vi "MID-VAC Timer.vi"(10 "TO sec (Start timer)":dbl format="%.2f", 11 "Action":T1) -> (3 "TO":bool)   [LabVIEW 2011]
uses:
  timerAction_typdef.ctl
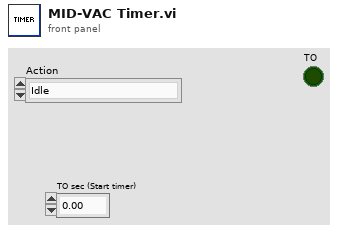
[diagram p1: front panel]
types:
  T1 = typedef "timerAction_typdef.ctl" = enum16{"Idle", "Start Timer", "Timer Running"}
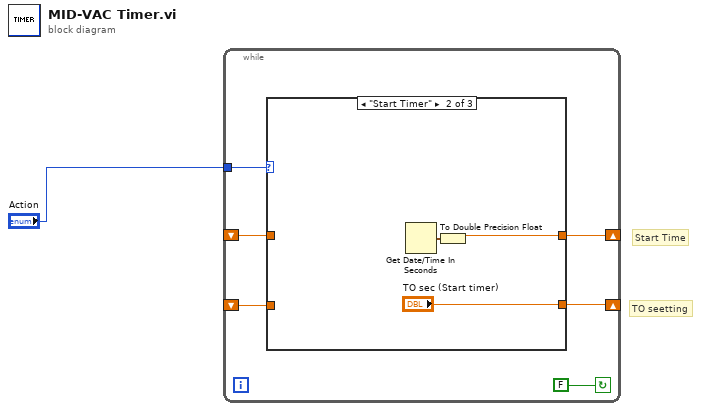
[diagram p0: block diagram]
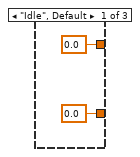
[diagram p2: hidden frame]
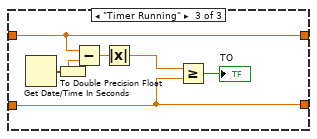
[diagram p3: hidden frame]
diagram:
  # "Start Time"
  # "TO seetting"
  n1 = while {
    tunnel: "Action" -> [w7]
    shift-right: [w6] -> _
    shift-left: _ -> [w3]
    shift-right: [w5] -> _
    shift-left: _ -> [w4]
    stop <- FALSE continue-if-true
    n2 = case shown="\"Start Timer\"" w7 {
      tunnel: [0.0 ("TO sec (Start timer)") "TO sec (Start timer)" w14] -> w6
      tunnel: [0.0 ("seconds since 1Jan1904") w11 w18] -> w5
      tunnel: w4 -> [_ _ w18]
      tunnel: w3 -> [_ _ w14]
      frame "Idle", Default {
      }
      frame "Start Timer" {
        n3 = Get Date/Time In Seconds() -> (seconds since 1Jan1904=w10:timestamp)
        n4 = To Double Precision Float(number=w10) -> (double precision float=w11:dbl)
      }
      frame "Timer Running" {
        n5 = Get Date/Time In Seconds() -> (seconds since 1Jan1904=w13:timestamp)
        n6 = To Double Precision Float(number=w13) -> (double precision float=w17:dbl)
        n7 = Subtract(x=w18, y=w17) -> (x-y=w16:dbl)
        n8 = Absolute Value(x=w16) -> (abs(x)=w15:dbl)
        n9 = Greater Or Equal?(x=w15, y=w14) -> (x >= y?=→"TO":bool)
      }
    }
  }
